vi "sub_main_statistics.vi"(8 "error in":errorcluster) -> (0 "error out":errorcluster)   [LabVIEW 2019]
uses:
  Ctrl/cmd_ini-RW.ctl
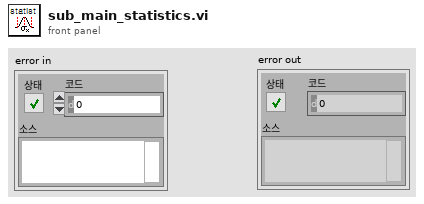
[diagram p1: front panel]
types:
  T1 = typedef "cmd_ini-RW.ctl" = enum16{"ini", "read", "write"}
  T2 = typedef "statistics_val.ctl" = cluster{"gap plus mean":dbl, "gap plus max":dbl, "gap plus sum":dbl, "gap minus mean":dbl, "gap minus max":dbl, "gap minus sum":dbl, "gap abs mean":dbl, "gap abs max":dbl, "gap abs sum":dbl, "wpt length":dbl, "total moving time":dbl, "average speed":dbl, "plus gap count":u64, "minus gap count":u64, "drive length":dbl}
  T3 = cluster{"total time":dbl, "run time":dbl, "wait time":dbl}
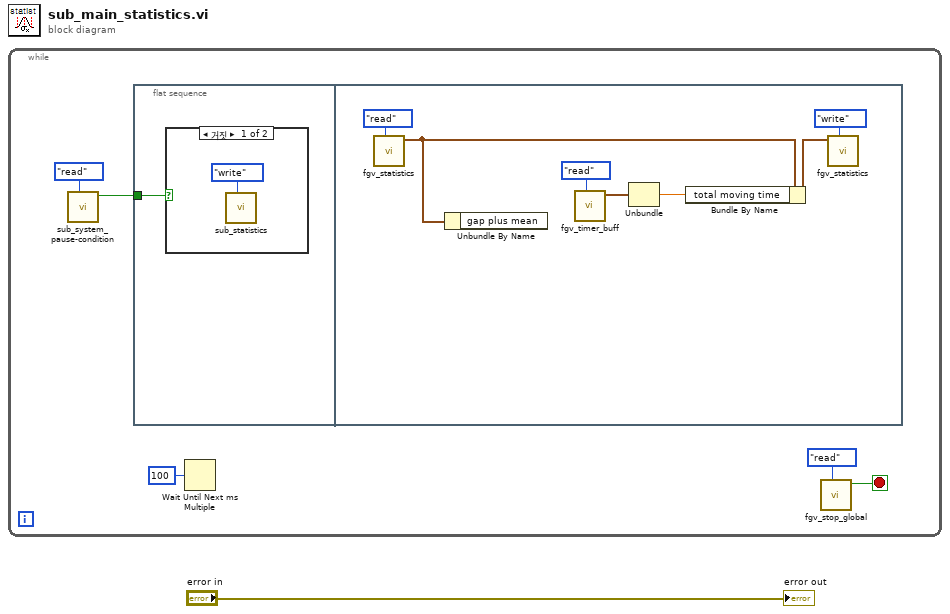
[diagram p0: block diagram]
diagram:
  n1 = while {
    stop <- w5 stop-if-true
    n2 = call "sub_system_pause-condition.vi"("cmd"=enum16{"pause", "go", "read"}."read") -> ("pause"=w2:bool)  [unwired: 10 in]
    n3 = flat-sequence {
      tunnel: w2 -> [w7]
      frame #0 {
        n4 = case shown="거짓" w7 {
          frame False {
            n5 = call "sub_statistics.vi"("cmd"=enum16{"ini", "read", "write"}."write") -> ()  [unwired: 10 in, 1 out]
          }
          frame True {
          }
        }
      }
      frame #1 {
        n6 = call "fgv_statistics.vi"("cmd"=cmd_ini-RW."read") -> ("statistics values out"=w9:T2)  [unwired: 10 in]
        n7 = Unbundle By Name(w9) -> ()  [unwired: 1 out]
        n8 = call "fgv_timer_buff.vi"("cmd"=enum16{"write", "read"}."read") -> ("time_status out"=w11:T3)  [unwired: 10 in]
        n9 = Unbundle(w11) -> ("run time"=w10:dbl)  [unwired: 2 out]
        n10 = Bundle By Name(cluster=w9, "total moving time"=w10) -> (w12:T2)
        n11 = call "fgv_statistics.vi"("cmd"=cmd_ini-RW."write", "statistics values"=w12) -> ()  [unwired: 9 in, 1 out]
      }
    }
    n12 = Wait Until Next ms Multiple(millisecond multiple=u32 100 ("ms 배수")) -> ()  [unwired: 1 out]
    n13 = call "fgv_stop_global.vi"("cmd"=enum16{"init", "stop", "read"}."read") -> ("val_out"=w5:bool)  [unwired: 10 in]
  }
  "error out" <- "error in"
